vi "Robot Global Data.vi"() -> ()   [LabVIEW 2018]
doc: "This global VI can contain as many global variables as you need. Place a control on the panel, give it a good name. To read or write to it from a VI, drag the icon to the diagram of that VI. You can also drag from the project. Click on the node to change which global you access. You shouldn't have multiple locations writing to a global or it will cause a race-condition."
uses:
  <vilib>/Rock Robotics/WPI/Camera/WPI_CameraImageSize.ctl
  <vilib>/Rock Robotics/WPI/DriverStation/WPI_DriverStationRobotMode2.ctl
  Swerve Drive/Vision Data.ctl
  Swerve Drive/Offsets.ctl
panel:
  in  "Hold Position":dbl
  in  "Hold Mode":bool
  in  "pivotEnc":dbl
  in  "Offsets":T1
  out "Auto Commands":bool[](array[boolean])
  out "Time Start":dbl
  out "Hit":bool
  out "Vision Data":T2
  in  "YRPHfH":T3
  in  "Robot Mode":T4
  in  "image size":T5=enum."320x240"
  in  "Enable Vision":bool
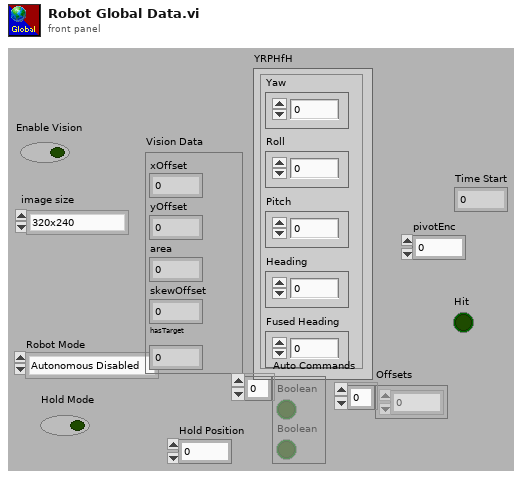
[diagram p1: front panel]
types:
  T1 = typedef "Offsets.ctl" = dbl[]
  T2 = typedef "Vision Data.ctl" = cluster{"xOffset":dbl, "yOffset":dbl, "area":dbl, "skewOffset":dbl, "hasTarget":dbl}
  T3 = cluster{"Yaw":dbl, "Roll":dbl, "Pitch":dbl, "Heading":dbl, "Fused Heading":dbl}
  T4 = typedef "WPI_DriverStationRobotMode2.ctl" = enum16{"Autonomous Disabled", "Autonomous Enabled", "Teleop Disabled", "Teleop Enabled", "Disconnected", "Finish", "Test Disabled", "Test Enabled", "Emergency Stopped"}
  T5 = typedef "WPI_CameraImageSize.ctl" = enum16{"640x480", "320x240", "160x120", "Custom"}
diagram:
